vi "Set Allow Echo Frames.vi"(8 "error in":errorcluster, 10 "Enable":bool, 11 "TPCANHandle in":T2=81 items=["PCAN_NONEBUS"=0, "PCAN_USBBUS1"=81, "PCAN_USBBUS2"=82, "PCAN_USBBUS3"=83, "PCAN_USBBUS4"=84, "PCAN_USBBUS5"=85, "PCAN_USBBUS6"=86, "PCAN_USBBUS7"=87, "PCAN_USBBUS8"=88, "PCAN_USBBUS9"=1289, "PCAN_USBBUS10"=1290, "PCAN_USBBUS11"=1291, "PCAN_USBBUS12"=1292, "PCAN_USBBUS13"=1293, "PCAN_USBBUS14"=1294, "PCAN_USBBUS15"=1295, "PCAN_USBBUS16"=1296]) -> (0 "error out":errorcluster, 3 "TPCANHandle out":T2=81 items=["PCAN_NONEBUS"=0, "PCAN_USBBUS1"=81, "PCAN_USBBUS2"=82, "PCAN_USBBUS3"=83, "PCAN_USBBUS4"=84, "PCAN_USBBUS5"=85, "PCAN_USBBUS6"=86, "PCAN_USBBUS7"=87, "PCAN_USBBUS8"=88, "PCAN_USBBUS9"=1289, "PCAN_USBBUS10"=1290, "PCAN_USBBUS11"=1291, "PCAN_USBBUS12"=1292, "PCAN_USBBUS13"=1293, "PCAN_USBBUS14"=1294, "PCAN_USBBUS15"=1295, "PCAN_USBBUS16"=1296], 5 "TPCANStatus":T1 items=["PCAN_ERROR_OK"=0, "PCAN_ERROR_XMTFULL"=1, "PCAN_ERROR_OVERRUN"=2, "PCAN_ERROR_BUSLIGHT"=4, "PCAN_ERROR_BUSHEAVY"=8, "PCAN_ERROR_BUSPASSIVE"=262144, "PCAN_ERROR_BUSOFF"=16, "PCAN_ERROR_QRCVEMPTY"=32, "PCAN_ERROR_QOVERRUN"=64, "PCAN_ERROR_QXMTFULL"=128, "PCAN_ERROR_REGTEST"=256, "PCAN_ERROR_NODRIVER"=512, "PCAN_ERROR_HWINUSE"=1024, "PCAN_ERROR_NETINUSE"=2048, "PCAN_ERROR_ILLHW"=5120, "PCAN_ERROR_ILLNET"=6144, "PCAN_ERROR_ILLCLIENT"=7168, "PCAN_ERROR_RESOURCE"=8192, "PCAN_ERROR_ILLPARAMTYPE"=16384, "PCAN_ERROR_ILLPARAMVAL"=32768, "PCAN_ERROR_UNKNOWN"=65536, "PCAN_ERROR_ILLDATA"=131072, "PCAN_ERROR_ILLMODE"=524288, "PCAN_ERROR_CAUTION"=33554432, "PCAN_ERROR_INITIALIZE"=67108864, "PCAN_ERROR_ILLOPERATION"=134217728])   [LabVIEW 2020, in "PCANBasic.lvlib"]
doc: "This parameter helps the user to allow / disallow the reception of echo messages within a\nPCAN-Channel, this is, the reception of frames sent by itself. This parameter doesn’t affect\nthe acceptance filter of the PCAN-Channel. Furthermore, other applications working with the\nsame PCAN-Hardware can individually configure the reception of echo frames.\nNote that disabling the PCAN_RECEIVE_STATUS parameter also suppresses the reception of\necho frames.\n\nPossible values: This parameter can have one of these values: PCAN_PARAMETER_OFF, PCAN_PARAMETER_ON. Note that other values will considered invalid. \n\nDefault value: Disabled (PCAN_PARAMETER_OFF). \n\nPCAN-Device: All PCAN devices (excluding PCAN_NONEBUS channel). \n\nREMARKS: Reseting the hardware has a duration of ~ 500 milliseconds. After receiving the PCAN_ERROR_BUSOFF error, an application should wait that time before trying to read or write again."
uses:
  PCANBasic.lvlib
  TPCANParameter.ctl
  TPCANHandle.ctl
  TPCANStatus.ctl
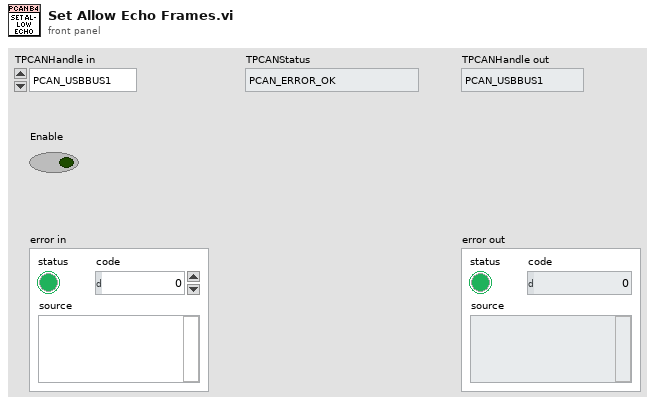
[diagram p1: front panel]
types:
  T1 = typedef "PCANBasic.lvlib/TPCANStatus.ctl" = u32
  T2 = typedef "PCANBasic.lvlib/TPCANHandle.ctl" = u16
  T3 = typedef "PCANBasic.lvlib/TPCANParameter.ctl" = enum8{"Unknown", "PCAN_DEVICE_ID", "PCAN_5VOLTS_POWER", "PCAN_RECEIVE_EVENT", "PCAN_MESSAGE_FILTER", "PCAN_API_VERSION", "PCAN_CHANNEL_VERSION", "PCAN_BUSOFF_AUTORESET", "PCAN_LISTEN_ONLY", "PCAN_LOG_LOCATION", "PCAN_LOG_STATUS", "PCAN_LOG_CONFIGURE", "PCAN_LOG_TEXT", "PCAN_CHANNEL_CONDITION", "PCAN_HARDWARE_NAME", "PCAN_RECEIVE_STATUS", "PCAN_CONTROLLER_NUMBER", "PCAN_TRACE_LOCATION", "PCAN_TRACE_STATUS", "PCAN_TRACE_SIZE", "PCAN_TRACE_CONFIGURE", "PCAN_CHANNEL_IDENTIFYING", "PCAN_CHANNEL_FEATURES", "PCAN_BITRATE_ADAPTING", "PCAN_BITRATE_INFO", "PCAN_BITRATE_INFO_FD", "PCAN_BUSSPEED_NOMINAL", "PCAN_BUSSPEED_DATA", "PCAN_IP_ADDRESS", "PCAN_LAN_SERVICE_STATUS", "PCAN_ALLOW_STATUS_FRAMES", "PCAN_ALLOW_RTR_FRAMES", "PCAN_ALLOW_ERROR_FRAMES", "PCAN_INTERFRAME_DELAY", "PCAN_ACCEPTANCE_FILTER_11BIT", "PCAN_ACCEPTANCE_FILTER_29BIT", "PCAN_IO_DIGITAL_CONFIGURATION", "PCAN_IO_DIGITAL_VALUE", "PCAN_IO_DIGITAL_SET", "PCAN_IO_DIGITAL_CLEAR", "PCAN_IO_ANALOG_VALUE", "PCAN_FIRMWARE_VERSION", "PCAN_ATTACHED_CHANNELS_COUNT", "PCAN_ATTACHED_CHANNELS", "PCAN_ALLOW_ECHO_FRAMES", "PCAN_DEVICE_PART_NUMBER", "PCAN_HARD_RESET_STATUS", "PCAN_LAN_CHANNEL_DIRECTION", "PCAN_DEVICE_GUID"}
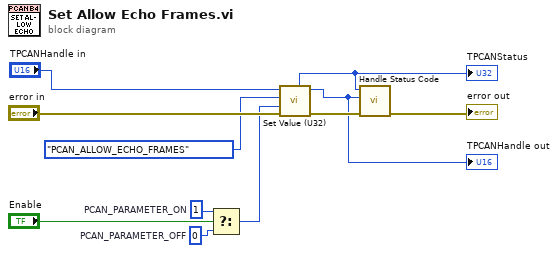
[diagram p0: block diagram]
diagram:
  w4 = u32 0  # PCAN_PARAMETER_OFF
  w5 = u32 1  # PCAN_PARAMETER_ON
  n1 = Select(t=w5, s="Enable", f=w4) -> (s? t:f=w3:u32)
  n2 = call "Set Value (U32).vi"("error in"="error in", "Value"=w3, "TPCANParameter"=TPCANParameter."PCAN_ALLOW_ECHO_FRAMES", "TPCANHandle in"="TPCANHandle in") -> ("error out"=w9:errorcluster, "TPCANHandle out"=w1:T2, "TPCANStatus"=w2:u32)  [unwired: 5 in]
  "TPCANHandle out" <- w1
  "TPCANStatus" <- w2
  n3 = call "Handle Status Code.vi"("error in"=w9, "TPCANHandle"=w1, "TPCANStatus"=w2) -> ("error out"=→"error out":errorcluster)  [unwired: 8 in]
